vi "mode1.vi"() -> ()   [LabVIEW 2018]
panel:
  in  "开关改变次数":dbl=31.0
  in  "频率改变次数":dbl=61.0
  in  "步进电机运动次数":dbl=41.0
  in  "确定按钮":bool
  in  "停止":bool
  in  "单片机串口":refnum<visa-resource-name>
  in  "步进电机串口":refnum<visa-resource-name>
  # "多频多角度模式"
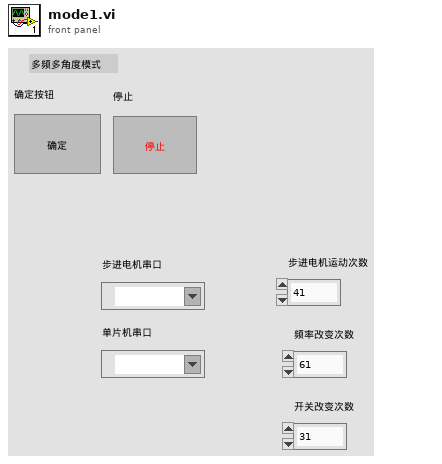
[diagram p1: front panel]
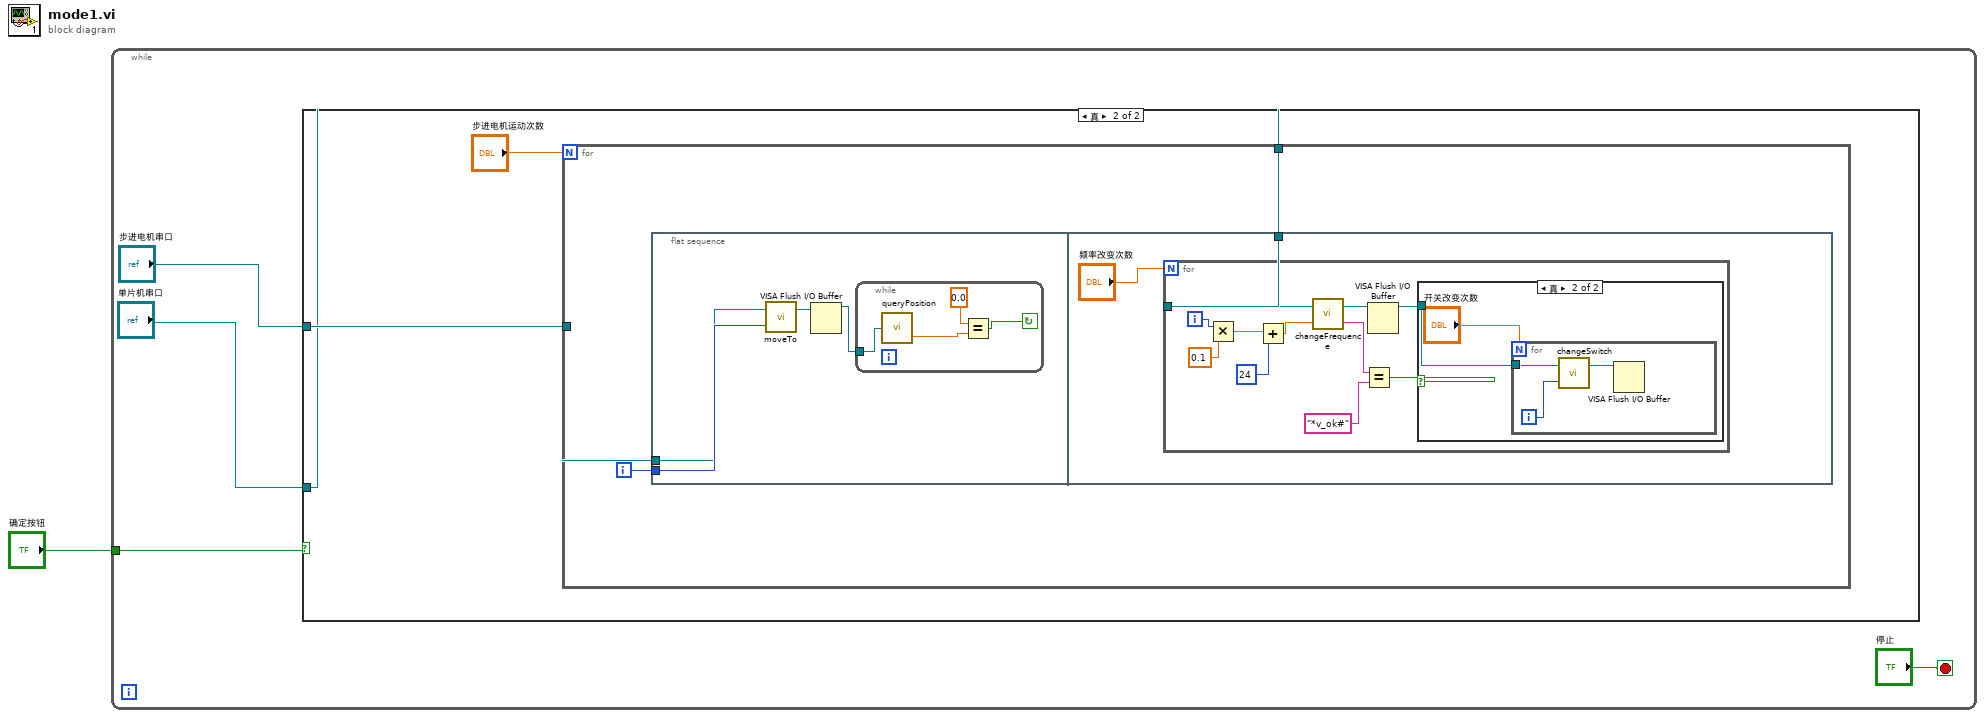
[diagram p0: block diagram]
diagram:
  n1 = while {
    tunnel: "确定按钮" -> [w4]
    stop <- "停止" stop-if-true
    n2 = case shown="真" w4 {
      tunnel: "步进电机串口" -> [_ w8]
      tunnel: "单片机串口" -> [_ w6]
      frame False {
      }
      frame True {
        n3 = for {
          N: "步进电机运动次数" -> [_]
          tunnel: w8 -> [w10]
          tunnel: w6 -> [w9]
          i -> [w11]
          n4 = flat-sequence {
            tunnel: w11 -> [w13]
            tunnel: w10 -> [w12]
            tunnel: w9 -> [w20]
            frame #0 {
              n5 = call "moveTo.vi"("移动到位置"=w13, "步进电机控制器串口"=w12) -> ("VISA资源名称"=w14:refnum<visa-resource-name>)  [unwired: 1 out]
              n6 = VISA Flush I/O Buffer(VISA resource name=w14) -> (VISA resource name out=w15:refnum<visa-resource-name>)  [unwired: 2 in, 1 out]
              n7 = while {
                tunnel: w15 -> [w16]
                stop <- w17 continue-if-true
                n8 = call "queryPosition.vi"("VISA资源名称"=w16) -> ("数值"=w19:dbl)  [unwired: 1 out]
                n9 = Equal?(x=0.0, y=w19) -> (x = y?=w17:bool)
              }
            }
            frame #1 {
              n10 = for {
                N: "频率改变次数" -> [_]
                tunnel: w20 -> [w23]
                i -> [w32]
                n11 = Multiply(x=w32, y=0.1) -> (x*y=w30:dbl)
                n12 = Add(x=w30, y=24) -> (x+y=w28:dbl)
                n13 = call "changeFrequence.vi"("频率值"=w28, "单片机串口"=w23) -> ("字符串"=w27:string, "单片机串口 2"=w24:refnum<visa-resource-name>)
                n14 = Equal?(x=w27, y="*v_ok#") -> (x = y?=w25:bool)
                n15 = VISA Flush I/O Buffer(VISA resource name=w24) -> (VISA resource name out=w22:refnum<visa-resource-name>)  [unwired: 2 in, 1 out]
                n16 = case shown="真" w25 {
                  tunnel: w22 -> [_ w34]
                  frame False {
                  }
                  frame True {
                    n17 = for {
                      N: "开关改变次数" -> [_]
                      tunnel: w34 -> [w35]
                      i -> [w37]
                      n18 = call "changeSwitch.vi"("数值"=w37, "单片机串口"=w35) -> ("单片机串口 2"=w36:refnum<visa-resource-name>)  [unwired: 1 out]
                      n19 = VISA Flush I/O Buffer(VISA resource name=w36) -> ()  [unwired: 2 in, 2 out]
                    }
                  }
                }
              }
            }
          }
        }
      }
    }
  }
